vi "SIWI_v1.0.vi"() -> ()   [LabVIEW 2018]
uses:
  <vilib>/Platform/TimedLoop/XDataNode/timing_clust.ctl
  <vilib>/Platform/TimedLoop/XDataNode/nitl_modes.ctl
  <vilib>/Platform/TimedLoop/XDataNode/wakeup.ctl
  <vilib>/DAQmx/read.llb/DAQmx Read (Analog 1D Wfm NChan NSamp).vi
  <vilib>/DAQmx/configure/timing.llb/DAQmx Timing (Sample Clock).vi
  <vilib>/DAQmx/miscellaneous.llb/DAQmx Fill In Error Info.vi
  <vilib>/platform/TimedLoop/XDataNode/XDataNode.xnode
  <vilib>/Platform/TimedLoop/XDataNode/XDNodeRunTimeDep.lvlib
  <resource>/objmgr/daqmx.rc
panel:
  in  "Gamry running":i32
  in  "Time between writeout (s)":dbl=10.0 min=0.0 step=1.0
  out "Running when lit for P, T below":bool
  out "Temperature":dbl caption="T (K)" format="%.2g"
  out "Pressure":dbl caption="P (MPa)" format="%.2g"
  out "Room temps":dynamicdata(graph)=[{"t0"=timestamp(3748813755.549279 s since 1904-01-01), "dt"=1.0, "Y"=[268.8098780241229]}, {"t0"=timestamp(3748813755.549279 s since 1904-01-01), "dt"=1.0, "Y"=[270.9771667325883]}, {"t0"=timestamp(3748813755.549279 s since 1904-01-01), "dt"=1.0, "Y"=[270.927425722561]}, {"t0"=timestamp(3748813755.549279 s since 1904-01-01), "dt"=1.0, "Y"=[270.0224537992005]}]
  in  "Time range for plots (h)":dbl=0.1 min=0.1 max=168.0 step=1.0 format="%.1f"
  in  "Clear plots":bool
  out "P2corr (MPa)":dbl=-724.982258450707
  out "P1corr (MPa)":dbl=-724.982258450707
  out "TC3 side":dbl=297.6006600731821
  out "TC2 PTD2":dbl=297.40935923692354
  out "TC1 top":dbl=297.37043318936816 caption="Numeric 7"
  out "TC0 bath":dbl=297.0570322976668
  out "RTD1 regressed T (K)":dbl=1558.4052872412326 format="%#_7g"
  out "RTD1 raw (Ohm)":dbl=499.679026164866 format="%#_8g"
  in  "Non-linearity_RTD1":dbl=0.1 format="%.6e"
  in  "C_RTD1":dbl=-1.087787e-12 format="%.6e"
  in  "B_RTD1":dbl=-5.998768e-07 format="%.6e"
  in  "A_RTD1":dbl=0.003912019 format="%.6e"
  in  "R0_RTD1 (at 0 C)":dbl=100.0231 format="%.6f"
  out "index":i32=1 caption="Index"
  in  "Tab":enum32{"Impedance", "Theta"}(tab)
  out "Impedance plot":cluster{dbl[], dbl[]}(graph)
  out "Phase plot":cluster{dbl[], dbl[]}(graph)
  out "Ph-a":dbl[](array[numeric]) caption="Theta (deg)" format="%_3g"
  out "Imp":dbl[](array[numeric]) caption="|Z| (ohm)"
  out "Freq":dbl[](array[numeric]) caption="Frequency"
  in  "Experiment description":string="Default"
  in  "testp":T1={"Start F"=1000000.0, "Stop F"=1000.0, "# Steps"=40, "Init Z guess (Ohm)"=10.0, "Device #"=0, "drv lvl"=0.01} caption="Gamry settings" {"drv lvl" min=0.001 max=0.1 step=0.001; "Device #" min=0 step=1; "Init Z guess (Ohm)" min=1 max=2000 format="%#_2g"; "# Steps" min=1 max=1800 step=1; "Stop F" min=1 max=3000000 step=1 format="%#_3f"; "Start F" min=20 max=3000000 step=1 format="%#_3f"}
  in  "Trigger Gamry sweep":bool
  in  "Halt":bool
  out "Pressures":dynamicdata(graph)=[{"t0"=timestamp(3748801016.0808024 s since 1904-01-01), "dt"=1.0, "Y"=[-336.9549373193859]}, {"t0"=timestamp(3748801016.0808024 s since 1904-01-01), "dt"=1.0, "Y"=[-337.2915207875254]}]
  out "P2raw (MPa)":dbl
  out "P2 corr to substract":dbl=105149.78666023392
  in  "aT (psi/K) 2":dbl=44.546 format="%#_13g"
  in  "T0_PTD2":dbl=297.647 format="%#_13g"
  out "P2corr (PSI)":dbl=-105149.78666023392
  out "P2raw (PSI)":dbl
  out "PTD currents":dynamicdata(graph)=[{"t0"=timestamp(3748801016.0808024 s since 1904-01-01), "dt"=1.0, "Y"=[-0.0020186692300000002]}, {"t0"=timestamp(3748801016.0808024 s since 1904-01-01), "dt"=1.0, "Y"=[-0.0011234076890000006]}] caption="Waveform Chart"
  out "PTD2 raw (mA)":dbl=3.9970561234140005e-06
  out "PTD1 raw (mA)":dbl=3.973899838370001e-06
  out "Base filename":string="20181115"
  in  "Root path":string="C:\\Users\\LAB319D\\gitHIPPOS\\calData\\"
  out "P1raw (MPa)":dbl
  out "P1 corr to substract":dbl=105149.78666023392
  in  "aT_PTD1 (PSI/K)":dbl=44.546 format="%#_13g"
  in  "T0_PTD1":dbl=297.647 format="%#_13g"
  out "P1corr (PSI)":dbl=-105149.78666023392
  out "Thermistor":waveform(dbl)(graph)={"t0"=timestamp(3748801016.0808024 s since 1904-01-01), "dt"=1.0, "Y"=[269.90040598743207]}
  out "DAQ cjtemp":dbl=299.38585358533464
  out "P1raw (PSI)":dbl
  out "Chamber temps":dynamicdata(graph)=[{"t0"=timestamp(3748801016.0808024 s since 1904-01-01), "dt"=1.0, "Y"=[268.77168263369003]}, {"t0"=timestamp(3748801016.0808024 s since 1904-01-01), "dt"=1.0, "Y"=[24.908036818797314]}, {"t0"=timestamp(3748801016.0808024 s since 1904-01-01), "dt"=1.0, "Y"=[270.9199737148546]}, {"t0"=timestamp(3748801016.0808024 s since 1904-01-01), "dt"=1.0, "Y"=[294.32974174548707]}]
  out "RTD raw R":dynamicdata(graph)=[{"t0"=timestamp(3748801016.0808024 s since 1904-01-01), "dt"=1.0, "Y"=[99.156546812277]}, {"t0"=timestamp(3748801016.0808024 s since 1904-01-01), "dt"=1.0, "Y"=[108.75600050222]}]
  out "RTD0 regressed T (K)":dbl=299.1672142593732 format="%#_7g"
  in  "Non-linearity_RTD0":dbl=0.1 format="%.6e"
  in  "C_RTD0":dbl=-2.572425e-12 format="%.6e"
  in  "B_RTD0":dbl=-5.972535e-07 format="%.6e"
  in  "A_RTD0":dbl=0.003912492 format="%.6e"
  out "RTD0 raw (Ohm)":dbl=110.16972814664 format="%#_8g"
  in  "R0_RTD0 (at 0 C)":dbl=100.0296 format="%.6f"
  # "Pressure measurement"
  # "MAIN CONTROLS"
  # "(no special characters)"
  # "Note: Do not halt run during Gamry sweep -- requires LabVIEW and Gamry reboot to correct."
  # "Conductivity measurement"
  # "Temperature measurement"
  # "RTD resistances"
  # "RTD calibration"
  # "Callendar - Van Dusen coefficients"
  # "Pressure transducer currents"
  # "PTD calibration"
  # "Reference coefficient 5.4545e-3"
  # "NI 9210 DAQ internal thermistor (calibration)"
  # "Temperature dependence\nreference coefficients\nT0 = 297.647 K\naT = 44.546 PSI/K"
  # "Calibration with ref. resistors"
  # "Standard CVD coefficients\nR0 = 100\nA = 3.9083e-3\nB = -5.775e-7\nC = 4.183e-12\n\nBURNS Engineering 927335\nR0 = 100.0259\nA = 3.914187e-3\nB = -6.266995e-7\nC = 1.161887e-11"
  # "CORR2: Linear dT between sample and reference\n(hotter thermocouple reads too hot)"
  # "CORR3: Linear dT between chamber and sensor\n(sensor outside of the sample chamber)\nTO BE ADJUSTED !!"
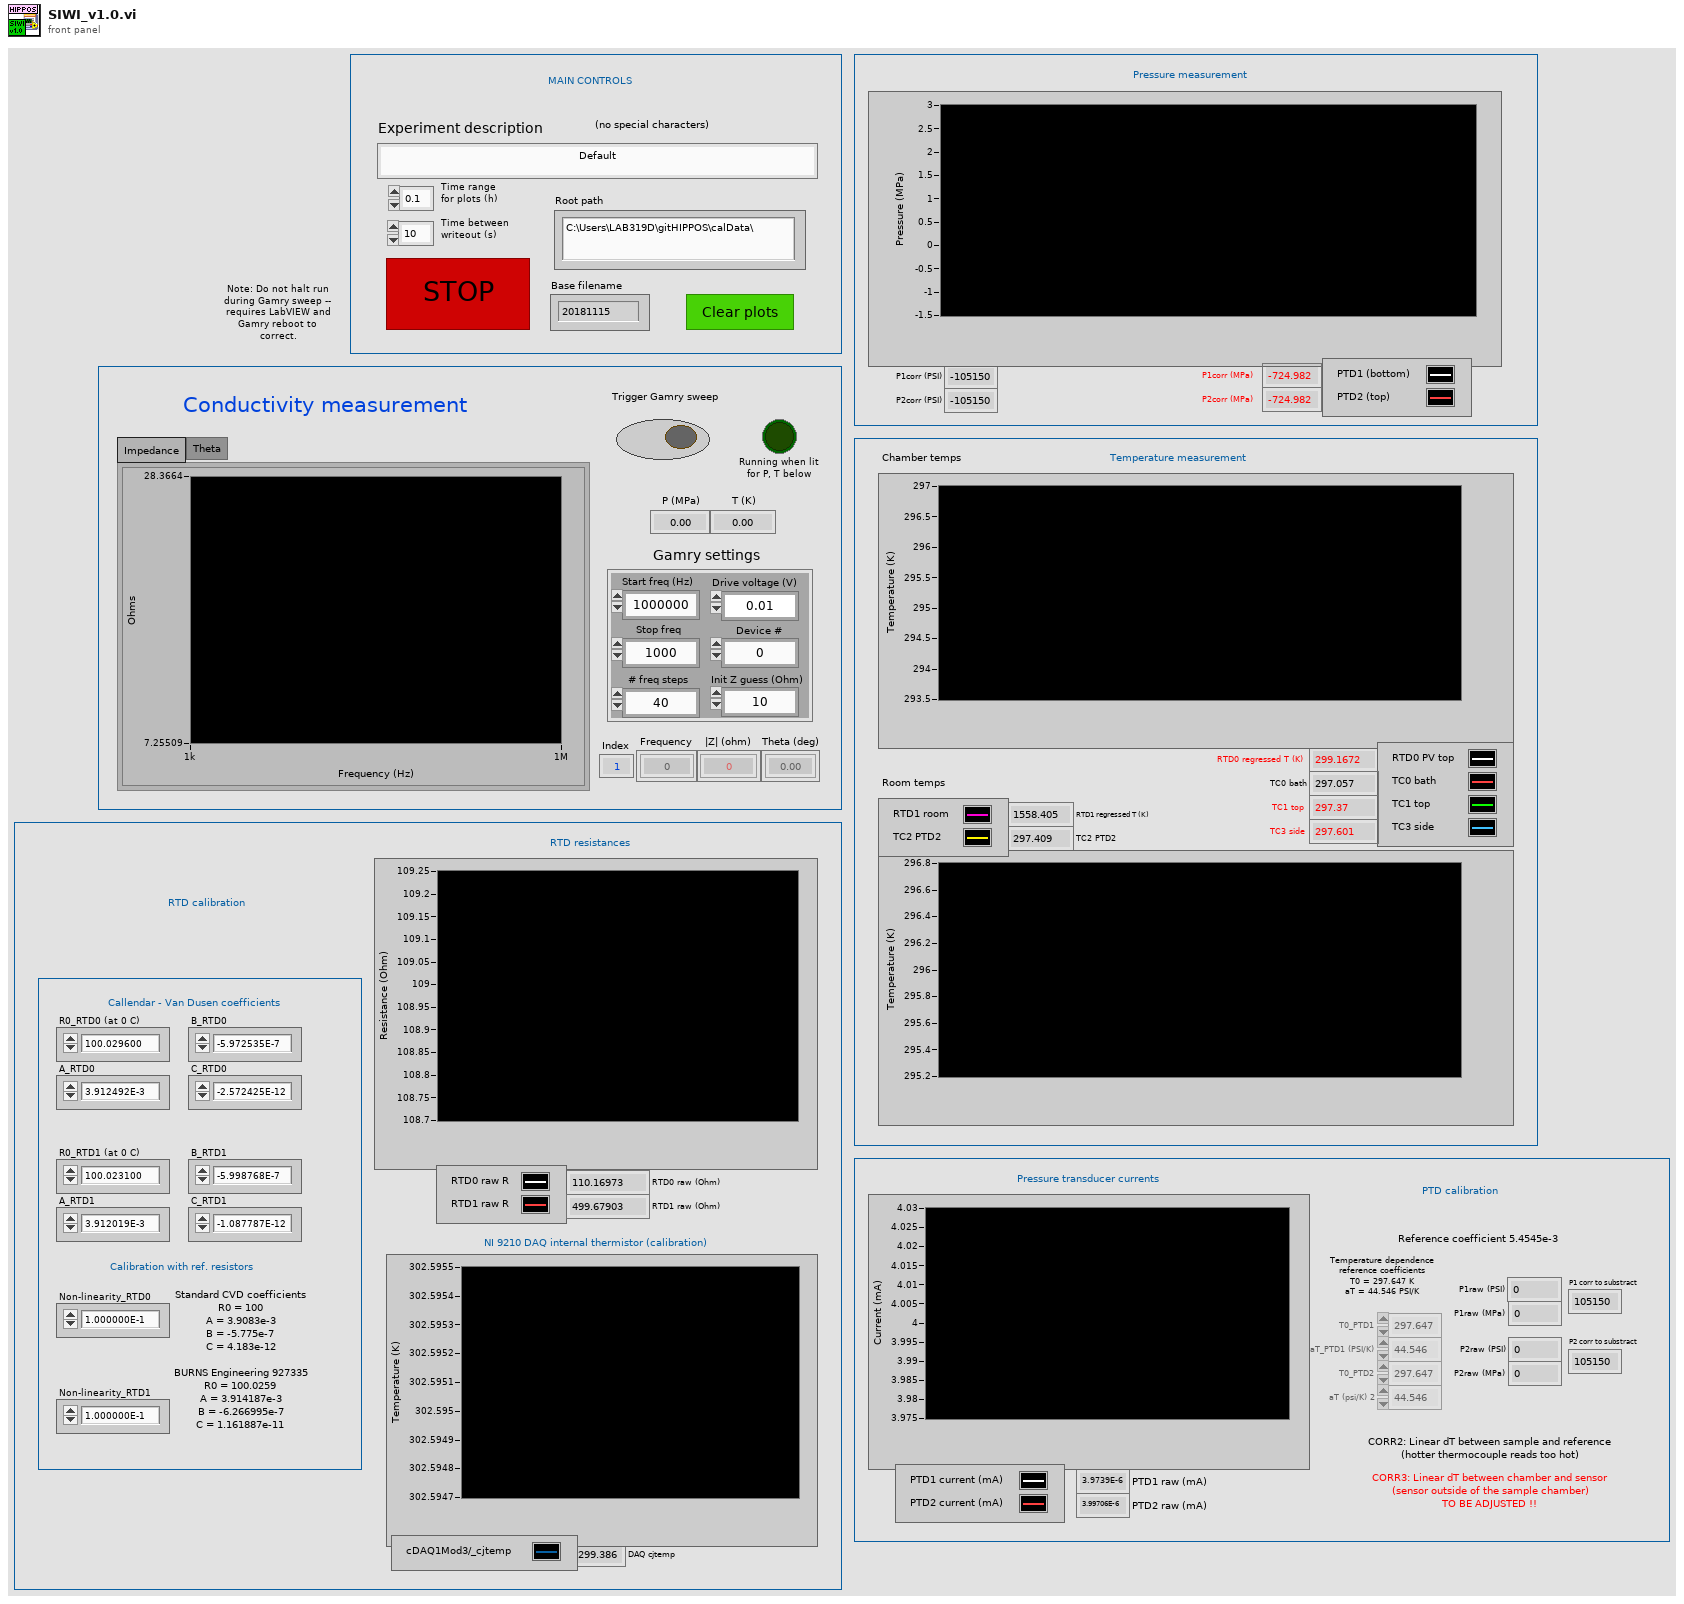
[diagram p1: front panel]
types:
  T1 = cluster{"Start F":sgl, "Stop F":sgl, "# Steps":u32, "Init Z guess (Ohm)":sgl, "Device #":i16, "drv lvl":sgl}
  T2 = enum16{"open", "replace", "create", "open or create", "replace or create", "replace or create with confirmation"}
  T3 = cluster{"refnum":refnum<file>, "P/T format string":string}
  T4 = cluster{"refnum":refnum<file>, "Cal format string":string}
  T5 = cluster{"dup path":path, "Experiment description":string, "Log file xtn":string}
  T6 = cluster{cluster{"refnum":refnum<file>, "Cal format string":string}, cluster{"refnum":refnum<file>, "P/T format string":string}, cluster{"dup path":path, "Experiment description":string, "Log file xtn":string}}
  T7 = typedef "XDNodeRunTimeDep.lvlib/timing_clust.ctl" = cluster{"Expected End [f-1]":u64, "Actual End [f-1]":u64, "Finished Late? [f-1]":bool, "Expected End [i-1]":u64, "Actual End [i-1]":u64, "Finished Late? [i-1]":bool, "Expected Start [i]":u64, "Actual Start [i]":u64, "Expected Start [f]":u64, "Actual Start [f]":u64, "Source Name":string, "Structure Name":string, "Period":i64, "Deadline":i64, "Offset":i64, "Start":i64, "Priority":i32, "Timeout":i32, "Mode":T8, "Wakeup Reason":T9, "Error":errorcluster, "Source Type":string, "Secondary Source Type":string, "Global End Time":u64, "Global Start Time":u64, "Frame Duration":u64, "Iteration Duration":u64, "Assigned CPU":i32, "I/O Scan Engine Mode":u32}
  T8 = typedef "XDNodeRunTimeDep.lvlib/nitl_modes.ctl" = enum32{"No Change", "Process missed periods, maintain original phase", "Discard missed periods, maintain original phase", "Process missed periods, ignore original phase", "Discard missed periods, ignore original phase"}
  T9 = typedef "XDNodeRunTimeDep.lvlib/wakeup.ctl" = enum32{"Normal", "Aborted", "Asynchronous wakeup", "Timing source error", "Timed loop error", "Timeout"}
  T10 = cluster{"T (K)":dbl, "T (K)":dbl, dbl, dbl, dbl, dbl}
  T11 = cluster{dbl, "T0_PTD1":dbl, "aT_PTD1 (PSI/K)":dbl, dbl}
  T12 = cluster{dbl, "T0_PTD2":dbl, "aT (psi/K) 2":dbl, dbl}
  T13 = cluster{"Imp":refnum<vi>, "Ph-a":refnum<vi>, "Freq":refnum<vi>}
  T14 = cluster{"Impedance plot":refnum<vi>, "Phase plot":refnum<vi>}
  T15 = cluster{cluster{"Imp":refnum<vi>, "Ph-a":refnum<vi>, "Freq":refnum<vi>}, cluster{"Impedance plot":refnum<vi>, "Phase plot":refnum<vi>}, "index":refnum<vi>}
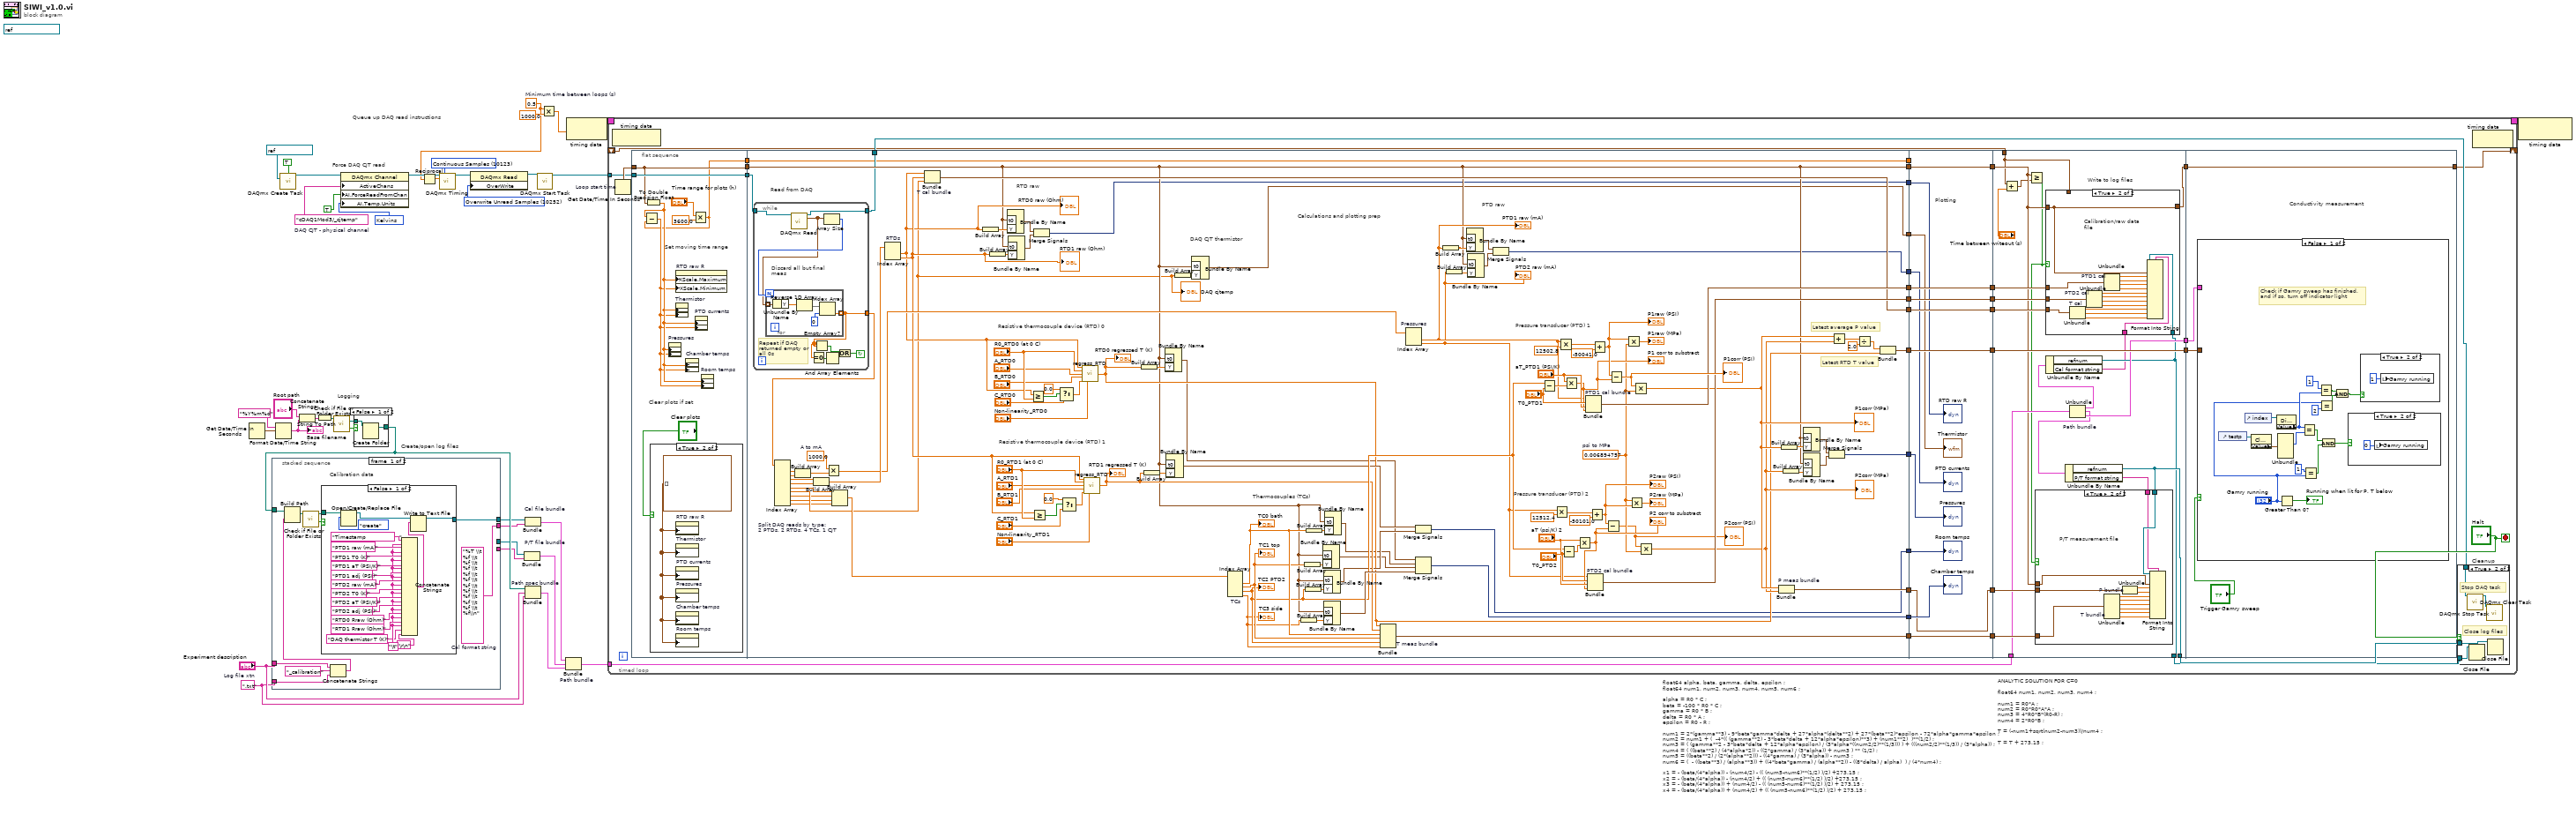
[diagram p0: block diagram]
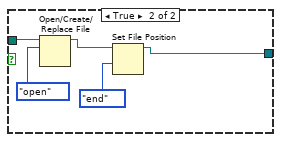
[diagram p2: hidden frame]
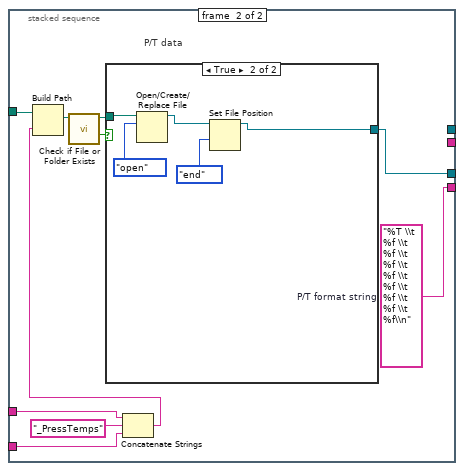
[diagram p3: hidden frame]
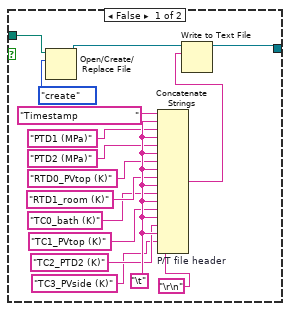
[diagram p4: hidden frame]
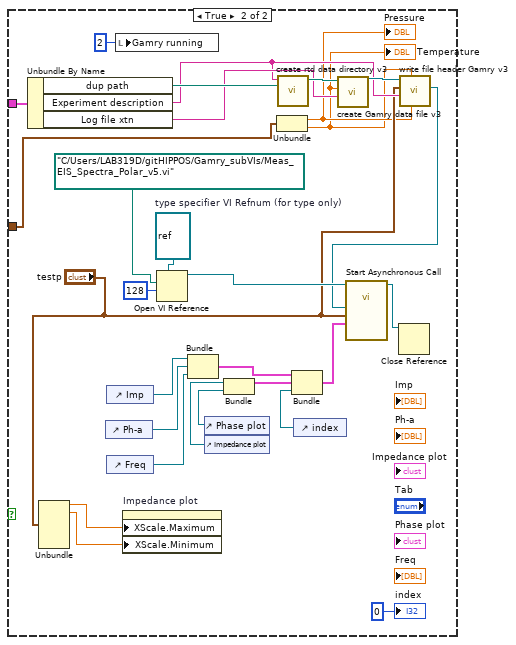
[diagram p12: hidden frame]
diagram:
  w4 = 10252 items=["Overwrite Unread Samples"=10252, "Do Not Overwrite Unread Samples"=10159] ("OverWrite")
  w5 = 10123 items=["Finite Samples"=10178, "Continuous Samples"=10123, "Hardware Timed Single Point"=12522] ("sample mode")
  w6 = 10325 items=["Deg C"=10143, "Deg F"=10144, "Kelvins"=10325, "Deg R"=10145, "From Custom Scale"=10065] ("AI.Temp.Units")
  w12 = tag "cDAQ1Mod3/_cjtemp"  # DAQ CJT - physical channel
  (unwired) refnum<k21> "MyVoltageTask"
  w23 = ".txt"  # Log file xtn
  w7 = 0.5  # Minimum time between loops (s)
  # "Force DAQ CJT read"
  # "Logging"
  # "Queue up DAQ read instructions"
  # "Create/open log files"
  # "ANALYTIC SOLUTION FOR C=0\n\nfloat64 num1, num2, num3, num4 ;\n\nnum1 = R0*A ;\nnum2 = R0*R0*A*A ;\nnum3 = 4*R0*B*(R0-R) ;\nnum4 = 2*R0*B ;\n\nT = (-num1+sqrt(num2-num3))/num4 ;\n\nT = T + 273.15 ;"
  # "float64 alpha, beta, gamma, delta, epsilon ;\nfloat64 num1, num2, num3, num4, num5, num6 ;\n\nalpha = R0 * C ;\nbeta = -100 * R0 * C ;\ngamma = R0 * B ;\ndelta = R0 * A ;\nepsilon = R0 - R ;\n\nnum1 = 2*(gamma**3) - 9*beta*gamma*delta + 27*alpha*(delta**2) + 27*(beta**2)*epsilon - 72*alpha*gamma*epsilon ;\nnum2 = num1 + (  -4*(( (gamma**2) - 3*beta*delta + 12*alpha*epsilon)**3) + (num1**2)  )**(1/2) ;\nnum3 = ( (gamma**2 - 3*beta*delta + 12*alpha*epsilon) / (3*alpha*((num2/2)**(1/3))) ) + (((num2/2)**(1/3)) / (3*alpha)) ;\nnum4 = ( ((beta**2) / (4*alpha*2)) - ((2*gamma) / (3*alpha)) + num3 ) ** (1/2) ;\nnum5 = ((beta**2) / (2*(alpha**2))) - ((4*gamma) / (3*alpha)) - num3 ;\nnum6 = (  - ((beta**3) / (alpha**3)) + ((4*beta*gamma) / (alpha**2)) - ((8*delta) / alpha)  ) / (4*num4) ;\n\nx1 = - (beta/(4*alpha)) - (num4/2) - (( (num5-num6)**(1/2) )/2) +273.15 ;\nx2 = - (beta/(4*alpha)) - (num4/2) + (( (num5-num6)**(1/2) )/2) +273.15 ;\nx3 = - (beta/(4*alpha)) + (num4/2) - (( (num5-num6)**(1/2) )/2) + 273.15 ;\nx4 = - (beta/(4*alpha)) + (num4/2) + (( (num5-num6)**(1/2) )/2) + 273.15 ;"
  n1 = Get Date/Time In Seconds() -> (seconds since 1Jan1904=w32:timestamp)
  n2 = Format Date/Time String(time format string (%c)="%Y%m%d", seconds (now)=w32) -> (date/time string=w26:string)  [unwired: 1 in]
  "Base filename" <- w26
  n3 = call <vilib>:"DAQmx Create Task.vi"("auto cleanup"=TRUE, "task to copy"=refnum<k21> "DAQreadAll") -> ("task out"=w10:refnum<k21>)  [unwired: 12 in, 1 out]
  n4 = Concatenate Strings("Root path", w26) -> (w30:string)
  n5 = String To Path(string=w30) -> (path=w29:path)
  n6 = call <vilib>:"Check if File or Folder Exists.vi"("path"=w29) -> ("file or folder exists?"=w27:bool, "dup path"=w28:path)  [unwired: 8 in, 1 out]
  n7 = property class="DAQmx Channel"(reference=w10, "ActiveChans"=w12, "AI.ForceReadFromChan"=TRUE, "AI.Temp.Units"=w6) -> (reference out=w9:refnum<k21>)  [unwired: 1 in, 1 out]
  n8 = case shown="False" w27 {
    tunnel: [w39 w40] -> w25
    tunnel: w28 -> [w38 w40]
    frame False {
      n9 = Create Folder(path (use dialog)=w38) -> (created path=w39:path)  [unwired: 2 in, 2 out]
    }
    frame True {
    }
  }
  n10 = stacked-sequence {
    tunnel: "Experiment description" -> [w49 w83]
    tunnel: w23 -> [w48 w82]
    tunnel: w25 -> [w44 w78]
    tunnel: [_ w76] -> w20
    tunnel: [_ w75] -> w19
    tunnel: [w42 _] -> w22
    tunnel: [w41 _] -> w21
    frame #0 {
      w41 = "%T \\t %f \\t %f \\t %f \\t %f \\t %f \\t %f \\t %f \\t %f \\t %f \\t %f \\t %f\\n"  # Cal format string
      # "Calibration data"
      n11 = Concatenate Strings(w49, "_calibration", w48) -> (w43:string)
      n12 = Build Path(base path=w44, name or relative path=w43) -> (appended path=w45:path)
      n13 = call <vilib>:"Check if File or Folder Exists.vi"("path"=w45) -> ("file or folder exists?"=w46:bool, "dup path"=w47:path)  [unwired: 8 in, 1 out]
      n14 = case shown="False" w46 {
        tunnel: w47 -> [w69 w74]
        tunnel: [w66 w70] -> w42
        frame False {
          w52 = "\t"
          n15 = Open/Create/Replace File(file path (use dialog)=w69, operation (0:open)=T2."create") -> (refnum out=w67:refnum<file>)  [unwired: 4 in, 2 out]
          n16 = Concatenate Strings("Timestamp                   " ("P/T file header"), w52, "PTD1 raw (mA)" ("P/T file header"), w52, "PTD1 T0 (K)" ("P/T file header"), w52, "PTD1 aT (PSI/K)" ("P/T file header"), w52, "PTD1 adj (PSI)" ("P/T file header"), w52, "PTD2 raw (mA)" ("P/T file header"), w52, "PTD2 T0 (K)" ("P/T file header"), w52, "PTD2 aT (PSI/K)" ("P/T file header"), w52, "PTD2 adj (PSI)" ("P/T file header"), w52, "RTD0 Rraw (Ohm)" ("P/T file header"), w52, "RTD1 Rraw (Ohm)" ("P/T file header"), w52, "DAQ thermistor T (K)" ("P/T file header"), "\r\n") -> (w54:string)
          n17 = Write to Text File(file (use dialog)=w67, text=w54) -> (refnum out=w66:refnum<file>)  [unwired: 2 in, 2 out]
        }
        frame True {
          n18 = Open/Create/Replace File(file path (use dialog)=w74, operation (0:open)=T2."open") -> (refnum out=w71:refnum<file>)  [unwired: 4 in, 2 out]
          n19 = Set File Position(refnum=w71, from (0:start)=enum16{"start", "end", "current"}."end") -> (refnum out=w70:refnum<file>)  [unwired: 2 in, 1 out]
        }
      }
    }
    frame #1 {
      w75 = "%T \\t %f \\t %f \\t %f \\t %f \\t %f \\t %f \\t %f \\t %f\\n"  # P/T format string
      # "P/T data"
      n20 = Concatenate Strings(w83, "_PressTemps", w82) -> (w77:string)
      n21 = Build Path(base path=w78, name or relative path=w77) -> (appended path=w79:path)
      n22 = call <vilib>:"Check if File or Folder Exists.vi"("path"=w79) -> ("file or folder exists?"=w80:bool, "dup path"=w81:path)  [unwired: 8 in, 1 out]
      n23 = case shown="True" w80 {
        tunnel: w81 -> [w100 w105]
        tunnel: [w97 w101] -> w76
        frame False {
          w96 = "\t"
          n24 = Open/Create/Replace File(file path (use dialog)=w100, operation (0:open)=T2."create") -> (refnum out=w98:refnum<file>)  [unwired: 4 in, 2 out]
          n25 = Concatenate Strings "P/T file header"("Timestamp                   " ("P/T file header"), w96, "PTD1 (MPa)" ("P/T file header"), w96, "PTD2 (MPa)" ("P/T file header"), w96, "RTD0_PVtop (K)" ("P/T file header"), w96, "RTD1_room (K)" ("P/T file header"), w96, "TC0_bath (K)" ("P/T file header"), w96, "TC1_PVtop (K)" ("P/T file header"), w96, "TC2_PTD2 (K)" ("P/T file header"), w96, "TC3_PVside (K)" ("P/T file header"), "\r\n") -> (w86:string)
          n26 = Write to Text File(file (use dialog)=w98, text=w86) -> (refnum out=w97:refnum<file>)  [unwired: 2 in, 2 out]
        }
        frame True {
          n27 = Open/Create/Replace File(file path (use dialog)=w105, operation (0:open)=T2."open") -> (refnum out=w102:refnum<file>)  [unwired: 4 in, 2 out]
          n28 = Set File Position(refnum=w102, from (0:start)=enum16{"start", "end", "current"}."end") -> (refnum out=w101:refnum<file>)  [unwired: 2 in, 1 out]
        }
      }
    }
  }
  n29 = Reciprocal(x=w7) -> (1/x=w8:dbl)
  n30 = call-poly <vilib>:"DAQmx Timing.vi"("task/channels in"=w9, "sample mode"=w5, "rate"=w8) -> ("task out"=w3:refnum<k21>)  [unwired: 11 in, 1 out]
  n31 = property class="DAQmx Read"(reference=w3, "OverWrite"=w4) -> (reference out=w2:refnum<k21>)  [unwired: 1 in, 1 out]
  n32 = Bundle "P/T file bundle"("refnum"=w20, "P/T format string"=w19) -> (w16:T3)  [unwired: 1 in]
  n33 = Bundle "Cal file bundle"("refnum"=w22, "Cal format string"=w21) -> (w15:T4)  [unwired: 1 in]
  n34 = Bundle "Path spec bundle"("dup path"=w25, "Experiment description"="Experiment description", "Log file xtn"=w23) -> (w17:T5)  [unwired: 1 in]
  n35 = call <vilib>:"DAQmx Start Task.vi"("task/channels in"=w2) -> ("task out"=w1:refnum<k21>)  [unwired: 13 in, 1 out]
  n36 = Multiply(x=w7, y=1000.0) -> (x*y=w34:dbl)
  n37 = Bundle "Path bundle"(w15, w16, w17) -> (w18:T6)  [unwired: 1 in]
  n38 = node-c288(w34) -> (w37:T7)
  n39 = timed-loop {
    timing: w37 -> [_]
    timing-out: [_] -> w36
    tunnel: w18 -> [w141]
    tunnel: w1 -> [w134]
    shift-right: [w129] -> _
    shift-left: _ -> [w128]
    stop <- "Halt" stop-if-true
    n40 = node-c288() -> ()  [unwired: 1 in, 1 out]
    n41 = Get Date/Time In Seconds "Loop start time"() -> (seconds since 1Jan1904=w137:timestamp)
    n42 = flat-sequence {
      tunnel: w134 -> [w153]
      tunnel: w137 -> [w151]
      tunnel: [w151] -> w133
      tunnel: [w153] -> w132
      tunnel: [w146] -> w112
      tunnel: [w247] -> w127
      tunnel: [w176] -> w125
      tunnel: [w246] -> w123
      tunnel: [w245] -> w121
      tunnel: [w241] -> w119
      tunnel: [w237] -> w117
      tunnel: [w236] -> w115
      tunnel: w133 -> [w176]
      tunnel: w132 -> [w165]
      tunnel: [w166] -> w131
      tunnel: [w161] -> w113
      tunnel: w112 -> [w161]
      tunnel: [w160] -> w111
      tunnel: [w159] -> w110
      tunnel: [w158] -> w109
      tunnel: [w157] -> w108
      tunnel: [w156] -> w107
      tunnel: [w155] -> w106
      tunnel: w127 -> [w289]
      tunnel: [w289] -> w126
      tunnel: w125 -> [w288]
      tunnel: [w288] -> w124
      tunnel: w123 -> [w277]
      tunnel: [w277] -> w122
      tunnel: w121 -> [w287]
      tunnel: [w287] -> w120
      tunnel: w119 -> [w286]
      tunnel: [w286] -> w118
      tunnel: w117 -> [w285]
      tunnel: [w285] -> w116
      tunnel: w115 -> [w284]
      tunnel: [w284] -> w114
      tunnel: w113 -> [_]
      tunnel: w111 -> [w283]
      tunnel: w110 -> [w282]
      tunnel: w109 -> [w281]
      tunnel: w108 -> [w280]
      tunnel: w107 -> [w279]
      tunnel: w106 -> [w278]
      tunnel: w141 -> [w303]
      tunnel: [w309] -> w140
      tunnel: w126 -> [w309]
      tunnel: w124 -> [w301]
      tunnel: w122 -> [w308]
      tunnel: w120 -> [w307]
      tunnel: w118 -> [w306]
      tunnel: w116 -> [w305]
      tunnel: w114 -> [w304]
      tunnel: [w302] -> w139
      tunnel: [w291] -> w135
      tunnel: [w293] -> w136
      tunnel: [w298] -> w130
      tunnel: w128 -> [w297]
      tunnel: w140 -> [w344]
      tunnel: w139 -> [w343]
      tunnel: [w341] -> w129
      tunnel: w130 -> [w341]
      frame #0 {
        # "Set moving time range"
        # "Clear plots if set"
        n43 = To Double Precision Float(number=w151) -> (double precision float=w148:dbl)
        n44 = case shown="True" "Clear plots" {
          frame False {
          }
          frame True {
            w154 = waveform(dbl)[] [] ("History Data")
            n45 = property on="RTD raw R" class="WFChart (strict)"("History Data"=w154) -> ()  [unwired: 2 in, 2 out]
            n46 = property on="Thermistor" class="WFChart (strict)"("History Data"=w154) -> ()  [unwired: 2 in, 2 out]
            n47 = property on="PTD currents" class="WFChart (strict)"("History Data"=w154) -> ()  [unwired: 2 in, 2 out]
            n48 = property on="Pressures" class="WFChart (strict)"("History Data"=w154) -> ()  [unwired: 2 in, 2 out]
            n49 = property on="Chamber temps" class="WFChart (strict)"("History Data"=w154) -> ()  [unwired: 2 in, 2 out]
            n50 = property on="Room temps" class="WFChart (strict)"("History Data"=w154) -> ()  [unwired: 2 in, 2 out]
          }
        }
        n51 = Multiply(x="Time range for plots (h)", y=3600.0 ("x")) -> (x*y=w146:dbl)
        n52 = Subtract(x=w148, y=w146) -> (x-y=w147:dbl)
        n53 = property on="Pressures" class="WFChart (strict)"("XScale.Maximum"=w148, "XScale.Minimum"=w147) -> ()  [unwired: 2 in, 2 out]
        n54 = property on="Thermistor" class="WFChart (strict)"("XScale.Maximum"=w148, "XScale.Minimum"=w147) -> ()  [unwired: 2 in, 2 out]
        n55 = property on="RTD raw R" class="WFChart (strict)"("XScale.Maximum"=w148, "XScale.Minimum"=w147) -> ()  [unwired: 2 in, 2 out]
        n56 = property on="Chamber temps" class="WFChart (strict)"("XScale.Maximum"=w148, "XScale.Minimum"=w147) -> ()  [unwired: 2 in, 2 out]
        n57 = property on="PTD currents" class="WFChart (strict)"("XScale.Maximum"=w148, "XScale.Minimum"=w147) -> ()  [unwired: 2 in, 2 out]
        n58 = property on="Room temps" class="WFChart (strict)"("XScale.Maximum"=w148, "XScale.Minimum"=w147) -> ()  [unwired: 2 in, 2 out]
      }
      frame #1 {
        w201 = 1000.0  # A to mA
        w183 = 0.006894757  # psi to MPa
        # "Read from DAQ"
        # "Resistive thermocouple device (RTD) 1"
        # "Pressure transducer (PTD) 2"
        # "Thermocouples (TCs)"
        # "PTD raw"
        # "RTD raw"
        # "DAQ CJT thermistor"
        # "Calculations and plotting prep"
        # "Latest RTD T value"
        # "Resistive thermocouple device (RTD) 0"
        # "Latest average P value"
        # "Pressure transducer (PTD) 1"
        n59 = while {
          tunnel: [w265] -> w167
          tunnel: w165 -> [w268]
          tunnel: [w269] -> w166
          stop <- w267 continue-if-true
          # "Repeat if DAQ returned empty or all 0s"
          # "Discard all but final meas"
          n60 = call-poly <vilib>:"DAQmx Read.vi"("task/channels in"=w268) -> ("task out"=w269:refnum<k21>, "data"=w270:waveform(dbl)[])  [unwired: 12 in, 1 out]
          n61 = Array Size(array=w270) -> (size(s)=w271:i32)
          n62 = for {
            N: w271 -> [_]
            tunnel: w270 -> [w276] mode=indexing
            tunnel: [w274] -> w265 mode=indexing
            n63 = Unbundle By Name(w276) -> ("Y"=w272:dbl[])
            n64 = Reverse 1D Array(array=w272) -> (reversed array=w273:dbl[])
            n65 = Index Array(array=w273, index=0) -> (element=w274:dbl)
          }
          n66 = Equal To 0?(x=w265) -> (x = 0?=w264:bool[])
          n67 = Empty Array?(array=w265) -> (empty?=w266:bool)
          n68 = And Array Elements(Boolean array=w264) -> (logical AND=w263:bool)
          n69 = Or(x=w266, y=w263) -> (x .or. y?=w267:bool)
        }
        n70 = Index Array "Split DAQ reads by type:\n2 PTDs, 2 RTDs, 4 TCs, 1 CJT"(array=w167) -> (element #1=w204:dbl, element #2=w203:dbl, element #3=w175:dbl, element #4=w174:dbl, element #5=w173:dbl, element #6=w171:dbl, element #7=w170:dbl, element #8=w169:dbl, element #9=w168:dbl)  [unwired: 9 in]
        "DAQ cjtemp" <- w171
        n71 = Build Array(w204, w203) -> (w172:dbl[])
        n72 = Build Array(w175, w174) -> (w207:dbl[])
        n73 = Multiply(x=w201, y=w172) -> (x*y=w202:dbl[])
        n74 = Build Array(w173, w170, w169, w168) -> (w206:dbl[])
        n75 = Index Array "RTDs"(array=w207) -> (element #1=w178:dbl, element #2=w179:dbl)  [unwired: 2 in]
        "RTD0 raw (Ohm)" <- w178
        "RTD1 raw (Ohm)" <- w179
        n76 = Bundle "T cal bundle"(w178, w179, w171) -> (w236:cluster{dbl, dbl, dbl})  [unwired: 1 in]
        n77 = Build Array(w178) -> (w213:dbl[])
        n78 = Build Array(w179) -> (w226:dbl[])
        n79 = Bundle By Name("t0"=w176, "Y"=w213) -> (w216:waveform(dbl))  [unwired: 1 in]
        n80 = Bundle By Name("t0"=w176, "Y"=w226) -> (w215:waveform(dbl))  [unwired: 1 in]
        n81 = Greater Or Equal?(x=w178, y="R0_RTD0 (at 0 C)") -> (x >= y?=w230:bool)
        n82 = Greater Or Equal?(x=w179, y="R0_RTD1 (at 0 C)") -> (x >= y?=w223:bool)
        n83 = Merge Signals(w216, w215) -> (w160:dynamicdata)
        n84 = Select(t=0.0, s=w230, f="C_RTD0") -> (s? t:f=w228:dbl)
        n85 = Select(t=0.0, s=w223, f="C_RTD1") -> (s? t:f=w221:dbl)
        n86 = call "regress_RTD.vi"("R (Ohm)"=w178, "R0 (Ohm)"="R0_RTD0 (at 0 C)", "A (K^-1)"="A_RTD0", "B (K^-2)"="B_RTD0", "C (K^-3)"=w228, "dev"="Non-linearity_RTD0") -> ("T (K)"=w177:dbl)  [unwired: 9 in]
        "RTD0 regressed T (K)" <- w177
        n87 = call "regress_RTD.vi"("R (Ohm)"=w179, "R0 (Ohm)"="R0_RTD1 (at 0 C)", "A (K^-1)"="A_RTD1", "B (K^-2)"="B_RTD1", "C (K^-3)"=w221, "dev"="Non-linearity_RTD1") -> ("T (K)"=w184:dbl)  [unwired: 9 in]
        "RTD1 regressed T (K)" <- w184
        n88 = Build Array(w177) -> (w227:dbl[])
        n89 = Build Array(w184) -> (w217:dbl[])
        n90 = Bundle By Name("t0"=w176, "Y"=w227) -> (w164:waveform(dbl))  [unwired: 1 in]
        n91 = Bundle By Name("t0"=w176, "Y"=w217) -> (w181:waveform(dbl))  [unwired: 1 in]
        n92 = Build Array(w171) -> (w214:dbl[])
        n93 = Bundle By Name("t0"=w176, "Y"=w214) -> (w159:waveform(dbl))  [unwired: 1 in]
        n94 = Index Array "TCs"(array=w206) -> (element #1=w205:dbl, element #2=w200:dbl, element #3=w199:dbl, element #4=w198:dbl)  [unwired: 4 in]
        "TC0 bath" <- w205
        "TC1 top" <- w200
        "TC2 PTD2" <- w199
        "TC3 side" <- w198
        n95 = Build Array(w198) -> (w209:dbl[])
        n96 = Build Array(w200) -> (w211:dbl[])
        n97 = Build Array(w199) -> (w210:dbl[])
        n98 = Build Array(w205) -> (w212:dbl[])
        n99 = Bundle By Name("t0"=w176, "Y"=w211) -> (w163:waveform(dbl))  [unwired: 1 in]
        n100 = Bundle By Name("t0"=w176, "Y"=w210) -> (w180:waveform(dbl))  [unwired: 1 in]
        n101 = Bundle By Name("t0"=w176, "Y"=w209) -> (w208:waveform(dbl))  [unwired: 1 in]
        n102 = Bundle By Name("t0"=w176, "Y"=w212) -> (w162:waveform(dbl))  [unwired: 1 in]
        n103 = Bundle "T meas bundle"("T (K)"=w177, "T (K)"=w184, w205, w200, w199, w198) -> (w245:T10)  [unwired: 1 in]
        n104 = Index Array "Pressures"(array=w202) -> (element #1=w194:dbl, element #2=w192:dbl)  [unwired: 2 in]
        "PTD1 raw (mA)" <- w194
        "PTD2 raw (mA)" <- w192
        n105 = Merge Signals(w181, w180) -> (w156:dynamicdata)
        n106 = Merge Signals(w164, w162, w163, w208) -> (w157:dynamicdata)
        n107 = Build Array(w194) -> (w195:dbl[])
        n108 = Build Array(w192) -> (w193:dbl[])
        n109 = Bundle By Name("t0"=w176, "Y"=w195) -> (w197:waveform(dbl))  [unwired: 1 in]
        n110 = Bundle By Name("t0"=w176, "Y"=w193) -> (w196:waveform(dbl))  [unwired: 1 in]
        n111 = Merge Signals(w197, w196) -> (w158:dynamicdata)
        n112 = Subtract(x=w199, y="T0_PTD1") -> (x-y=w254:dbl)
        n113 = Multiply(x=w192, y=12512.4) -> (x*y=w260:dbl)
        n114 = Multiply(x=w194, y=12502.8) -> (x*y=w256:dbl)
        n115 = Subtract(x=w199, y="T0_PTD2") -> (x-y=w250:dbl)
        n116 = Multiply(x="aT_PTD1 (PSI/K)", y=w254) -> (x*y=w242:dbl)
        "P1 corr to substract" <- w242
        n117 = Multiply(x="aT (psi/K) 2", y=w250) -> (x*y=w238:dbl)
        "P2 corr to substract" <- w238
        n118 = Bundle "PTD1 cal bundle"(w194, "T0_PTD1"="T0_PTD1", "aT_PTD1 (PSI/K)"="aT_PTD1 (PSI/K)", w242) -> (w241:T11)  [unwired: 1 in]
        n119 = Bundle "PTD2 cal bundle"(w192, "T0_PTD2"="T0_PTD2", "aT (psi/K) 2"="aT (psi/K) 2", w238) -> (w237:T12)  [unwired: 1 in]
        n120 = Add(x=w260, y=-50101.0) -> (x+y=w251:dbl)
        "P2raw (PSI)" <- w251
        n121 = Add(x=w256, y=-50041.0) -> (x+y=w252:dbl)
        "P1raw (PSI)" <- w252
        n122 = Subtract(x=w251, y=w238) -> (x-y=w182:dbl)
        "P2corr (PSI)" <- w182
        n123 = Subtract(x=w252, y=w242) -> (x-y=w253:dbl)
        "P1corr (PSI)" <- w253
        n124 = Multiply(x=w252, y=w183) -> (x*y=→"P1raw (MPa)":dbl)
        n125 = Multiply(x=w183, y=w251) -> (x*y=→"P2raw (MPa)":dbl)
        n126 = Multiply(x=w253, y=w183) -> (x*y=w186:dbl)
        "P1corr (MPa)" <- w186
        n127 = Multiply(x=w182, y=w183) -> (x*y=w185:dbl)
        "P2corr (MPa)" <- w185
        n128 = Bundle "P meas bundle"(w186, w185) -> (w246:cluster{dbl, dbl})  [unwired: 1 in]
        n129 = Build Array(w186) -> (w188:dbl[])
        n130 = Build Array(w185) -> (w189:dbl[])
        n131 = Bundle By Name("t0"=w176, "Y"=w188) -> (w191:waveform(dbl))  [unwired: 1 in]
        n132 = Bundle By Name("t0"=w176, "Y"=w189) -> (w190:waveform(dbl))  [unwired: 1 in]
        n133 = Merge Signals(w191, w190) -> (w155:dynamicdata)
        n134 = Add(x=w186, y=w185) -> (x+y=w187:dbl)
        n135 = Divide(x=w187, y=2.0) -> (x/y=w248:dbl)
        n136 = Bundle(w248, "T (K)"=w177) -> (w247:cluster{dbl, "T (K)":dbl})  [unwired: 1 in]
      }
      frame #2 {
        # "Plotting"
        "RTD raw R" <- w283
        "Thermistor" <- w282
        "PTD currents" <- w281
        "Chamber temps" <- w280
        "Room temps" <- w279
        "Pressures" <- w278
      }
      frame #3 {
        # "Write to log files"
        n137 = Add(x=w297, y="Time between writeout (s)") -> (x+y=w300:timestamp)
        n138 = Greater Or Equal?(x=w301, y=w300) -> (x >= y?=w299:bool)
        n139 = Unbundle "Path bundle"(w303) -> (w292:T4, w295:T3, w302:T5)
        n140 = Unbundle By Name(w292) -> ("refnum"=w291:refnum<file>, "Cal format string"=w290:string)
        n141 = case shown="True" w299 {
          tunnel: w306 -> [_ w340]
          tunnel: w305 -> [_ w335]
          tunnel: w304 -> [_ w330]
          tunnel: w301 -> [_ w326]
          tunnel: [w323 w326] -> w298
          tunnel: w297 -> [w323 _]
          tunnel: w291 -> [_ w325]
          tunnel: w290 -> [_ w324]
          frame False {
          }
          frame True {
            # "Calibration/raw data file"
            n142 = Unbundle "T cal"(w330) -> (w329:dbl, w328:dbl, w327:dbl)
            n143 = Unbundle "PTD2 cal"(w335) -> (w334:dbl, "T0_PTD2"=w333:dbl, "aT (psi/K) 2"=w332:dbl, w331:dbl)
            n144 = Unbundle "PTD1 cal"(w340) -> (w339:dbl, "T0_PTD1"=w338:dbl, "aT_PTD1 (PSI/K)"=w337:dbl, w336:dbl)
            n145 = Format Into String(format string=w324, initial string=w325, w326, w339, w338, w337, w336, w334, w333, w332, w331, w329, w328, w327) -> ()  [unwired: 1 in, 2 out]
          }
        }
        n146 = Unbundle By Name(w295) -> ("refnum"=w293:refnum<file>, "P/T format string"=w294:string)
        n147 = case shown="True" w299 {
          tunnel: w308 -> [_ w322]
          tunnel: w307 -> [_ w319]
          tunnel: w301 -> [_ w312]
          tunnel: w294 -> [_ w310]
          tunnel: w293 -> [_ w311]
          frame False {
          }
          frame True {
            # "P/T measurement file"
            n148 = Unbundle "T bundle"(w319) -> ("T (K)"=w318:dbl, "T (K)"=w317:dbl, w316:dbl, w315:dbl, w314:dbl, w313:dbl)
            n149 = Unbundle "P bundle"(w322) -> (w321:dbl, w320:dbl)
            n150 = Format Into String(format string=w310, initial string=w311, w312, w321, w320, w318, w317, w316, w315, w314, w313) -> ()  [unwired: 1 in, 2 out]
          }
        }
      }
      frame #4 {
        # "Conductivity measurement"
        n151 = case shown="False" "Trigger Gamry sweep" {
          tunnel: w344 -> [_ w379]
          tunnel: w343 -> [_ w378]
          frame False {
            # "Check if Gamry sweep has finished,\nand if so, turn off indicator light"
            n152 = control-ref of="testp"() -> (w358:refnum<vi>)
            n153 = control-ref of="index"() -> (w357:refnum<vi>)
            n154 = property class="Clust (strict)"(reference=w358) -> ("Value"=w359:T1)  [unwired: 1 in, 2 out]
            n155 = property class="DigNum (strict)"(reference=w357) -> ("Value"=w352:i32)  [unwired: 1 in, 2 out]
            n156 = Unbundle(w359) -> ("# Steps"=w360:u32)  [unwired: 5 out]
            n157 = Greater Than 0?(x="Gamry running") -> (x > 0?=→"Running when lit for P, T below":bool)
            n158 = Equal?(x=w352, y=w360) -> (x = y?=w356:bool)
            n159 = Equal?(x=1, y="Gamry running") -> (x = y?=w354:bool)
            n160 = Equal?(x=1, y=w352) -> (x = y?=w347:bool)
            n161 = Equal?(x="Gamry running", y=2) -> (x = y?=w346:bool)
            n162 = And(x=w356, y=w354) -> (x .and. y?=w350:bool)
            n163 = And(x=w347, y=w346) -> (x .and. y?=w345:bool)
            n164 = case shown="True" w350 {
              frame False {
              }
              frame True {
                n165 = local write "Gamry running"(0 ("Gamry running")) -> ()
              }
            }
            n166 = case shown="True" w345 {
              frame False {
              }
              frame True {
                n167 = local write "Gamry running"(1 ("Gamry running")) -> ()
              }
            }
          }
          frame True {
            w385 = refnum<vi> refnum  # type specifier VI Refnum (for type only)
            n168 = Unbundle By Name(w378) -> ("dup path"=w377:path, "Experiment description"=w375:string, "Log file xtn"=w376:string)
            n169 = Unbundle("testp") -> ("Start F"=w367:sgl, "Stop F"=w368:sgl)  [unwired: 4 out]
            n170 = control-ref of="Ph-a"() -> (w370:refnum<vi>)
            n171 = control-ref of="Imp"() -> (w371:refnum<vi>)
            n172 = control-ref of="Freq"() -> (w372:refnum<vi>)
            n173 = local write "Gamry running"(2 ("Gamry running")) -> ()
            n174 = property on="Impedance plot" class="XYGraph (strict)"("XScale.Maximum"=w367, "XScale.Minimum"=w368) -> ()  [unwired: 2 in, 2 out]
            n175 = Open VI Reference(type specifier VI Refnum (for type only)=w385, vi path=path "C:/Users/LAB319D/gitHIPPOS/Gamry_subVIs/Meas_EIS_Spectra_Polar_v5.vi", options=128) -> (vi reference=w384:refnum<vi>)  [unwired: 3 in, 1 out]
            n176 = Bundle("Imp"=w371, "Ph-a"=w370, "Freq"=w372) -> (w390:T13)  [unwired: 1 in]
            n177 = control-ref of="Phase plot"() -> (w391:refnum<vi>)
            n178 = control-ref of="Impedance plot"() -> (w380:refnum<vi>)
            n179 = Bundle("Impedance plot"=w380, "Phase plot"=w391) -> (w389:T14)  [unwired: 1 in]
            n180 = Unbundle(w379) -> (w366:dbl, "T (K)"=w365:dbl)
            "Pressure" <- w366
            "Temperature" <- w365
            n181 = call "create rtd data directory v3.vi"("Base path"=w377, "description"=w375) -> ("dir path"=w381:path)  [unwired: 4 in, 1 out]
            n182 = control-ref of="index"() -> (w373:refnum<vi>)
            n183 = Bundle(w390, w389, "index"=w373) -> (w383:T15)  [unwired: 1 in]
            n184 = call "create Gamry data file v3.vi"("Extension"=w376, "temp"=w365, "dir path"=w381) -> ("refnum out"=w388:refnum<file>)  [unwired: 1 in, 3 out]
            n185 = call "write file header Gamry v3.vi"("Chamber pressure (MPa)"=w366, "Chamber temp (K)"=w365, "Description"=w375, "testp"="testp", "Output refnum"=w388) -> ("Refnum out"=w374:refnum<file>)  [unwired: 3 in, 1 out]
            n186 = call-by-ref "Start Asynchronous Call"(reference=w384, "output cluster"=w383, "testp"="testp", "Output file refnum"=w374) -> (reference out=w382:refnum<vi>)  [unwired: 10 in, 1 out]
            n187 = Close Reference(reference=w382) -> ()  [unwired: 1 in, 1 out]
            "index" <- 0
          }
        }
      }
    }
    n188 = case "Cleanup" shown="True" "Halt" {
      tunnel: w136 -> [_ w144]
      tunnel: w135 -> [_ w145]
      tunnel: w131 -> [_ w142]
      frame False {
      }
      frame True {
        # "Close log files"
        # "Stop DAQ task"
        n189 = call <vilib>:"DAQmx Stop Task.vi"("task/channels in"=w142) -> ("task out"=w143:refnum<k21>)  [unwired: 13 in, 1 out]
        n190 = Close File ("Close log files")(refnum=w145) -> ()  [unwired: 1 in, 2 out]
        n191 = call <vilib>:"DAQmx Clear Task.vi"("task in"=w143) -> ()  [unwired: 14 in, 1 out]
        n192 = Close File(refnum=w144) -> ()  [unwired: 1 in, 2 out]
      }
    }
    n193 = node-c288() -> ()  [unwired: 1 in, 1 out]
  }
  n194 = node-c288(w36) -> ()  [unwired: 1 out]
